vi "meTEC_Set_ID 50002_Live Set Voltage.vi"(6 "Instance (1)":u8=1, 8 "error in (no error)":errorcluster, 9 "TEC Configuration_IN":T1={"VISA resource name"="", "Device Address"=2}, 10 "Sequence No.":u16=5552, 11 "Live Set Voltage [V]":dbl) -> (0 "error out":errorcluster, 1 "TEC Configuration_OUT":T1={"VISA resource name"="", "Device Address"=2}, 3 "Serial Message_Read":string)   [LabVIEW 2023]
uses:
  TypeDefs/meTEC_Configuration.ctl
panel:
  # "--- Inputs ---"
  # "--- Outputs ---"
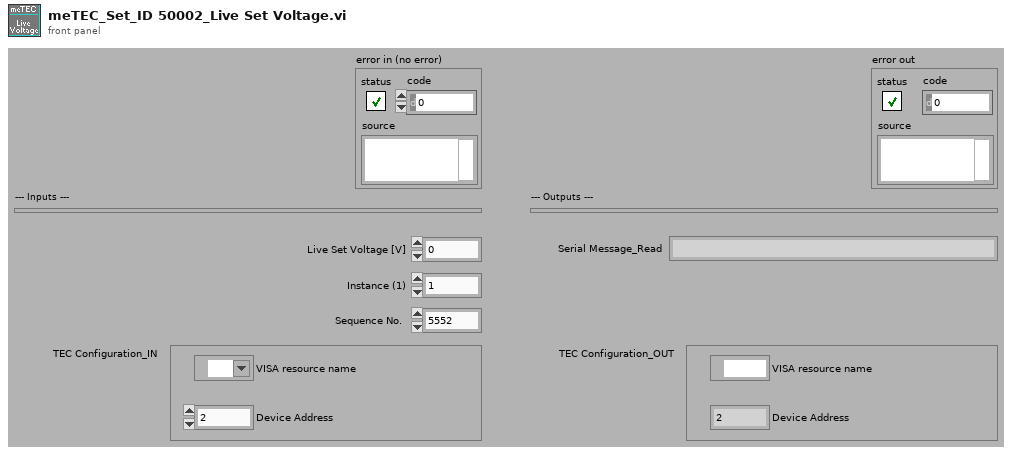
[diagram p1: front panel]
types:
  T1 = typedef "meTEC_Configuration.ctl" = cluster{"VISA resource name":refnum<visa-resource-name>, "Device Address":u16}
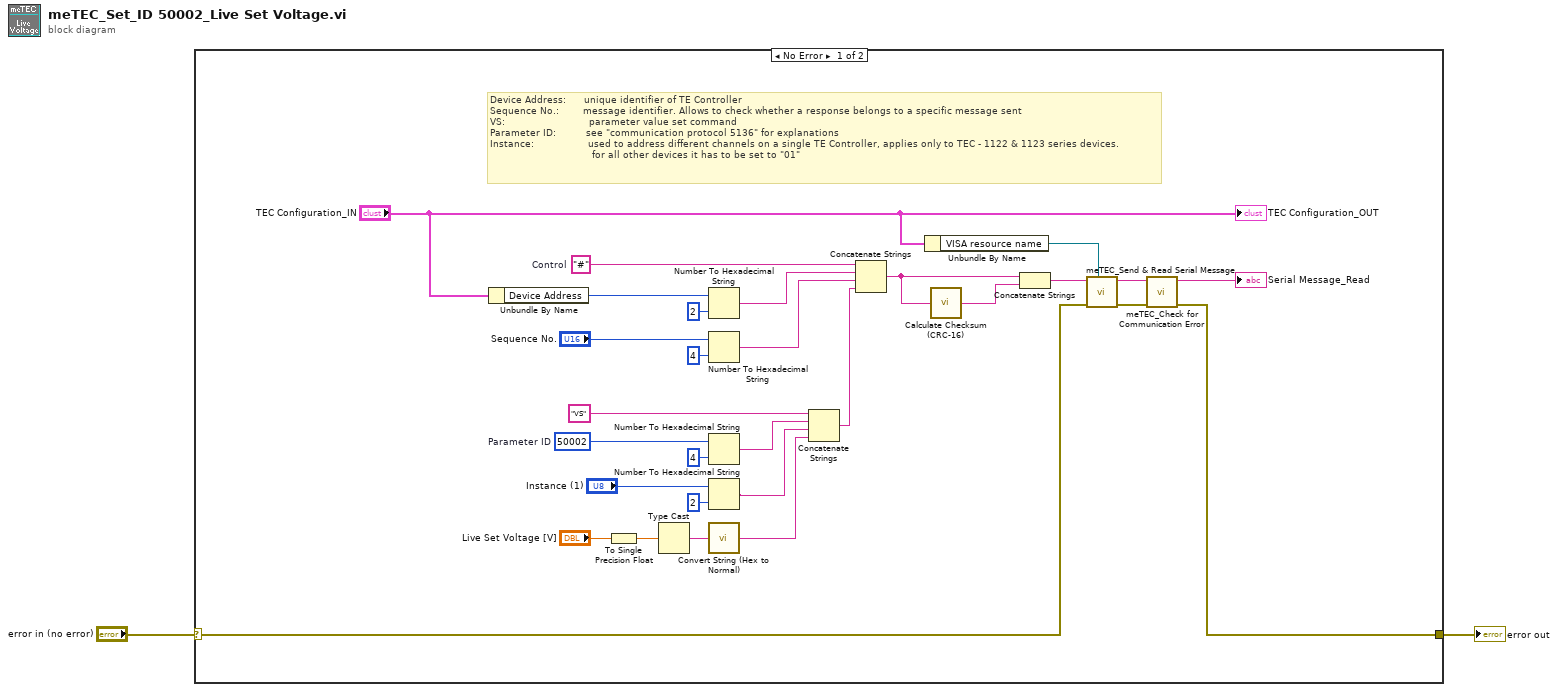
[diagram p0: block diagram]
diagram:
  n1 = case shown="No Error" "error in (no error)" {
    selector: "error in (no error)" -> [w15 w32]
    tunnel: [w5 w32] -> w2
    frame No Error {
      w23 = "#"  # Control
      w30 = 50002  # Parameter ID
      # "Device Address:      unique identifier of TE Controller\nSequence No.:        message identifier. Allows to check whether a response belongs to a specific message sent \nVS:                            parameter value set command\nParameter ID:          see \"communication protocol 5136\" for explanations\nInstance:                  used to address different channels on a single TE Controller, applies only to TEC - 1122 & 1123 series devices.\n                                  for all other devices it has to be set to \"01\""
      n2 = Unbundle By Name("TEC Configuration_IN") -> ("Device Address"=w10:u16)
      n3 = To Single Precision Float(number="Live Set Voltage [V]") -> (single precision float=w6:sgl)
      n4 = Type Cast(x=w6) -> (*(type *) &x=w26:string)  [unwired: 1 in]
      n5 = Number To Hexadecimal String(1:i16 2 ("width (-)"), 2:w10) -> (0:w18:string)
      n6 = Number To Hexadecimal String(1:i16 4 ("width (-)"), 2:"Sequence No.") -> (0:w22:string)
      n7 = Number To Hexadecimal String(1:i16 4 ("width (-)"), 2:w30) -> (0:w28:string)
      n8 = Number To Hexadecimal String(1:i16 2 ("width (-)"), 2:"Instance (1)") -> (0:w11:string)
      n9 = call "Convert String (Hex to Normal).vi"("Hex String"=w26) -> ("Normal String"=w27:string)  [unwired: 1 in]
      n10 = Concatenate Strings("VS", w28, w11, w27) -> (w17:string)
      n11 = Concatenate Strings(w23, w18, w22, w17) -> (w21:string)
      n12 = Unbundle By Name("TEC Configuration_IN") -> ("VISA resource name"=w13:refnum<visa-resource-name>)
      n13 = call "Calculate Checksum (CRC-16).vi"("Message"=w21) -> ("CRC [String]"=w20:string)  [unwired: 1 in]
      n14 = Concatenate Strings(w21, w20) -> (w16:string)
      n15 = call "meTEC_Send & Read Serial Message.vi"("VISA resource name"=w13, "error in (no error)"=w15, "Serial Message"=w16) -> ("error out"=w14:errorcluster, "Serial Message_Read"=w4:string)  [unwired: 7 in]
      n16 = call "meTEC_Check for Communication Error.vi"("error in (no error)"=w14, "Serial Message_IN"=w4) -> ("error out"=w5:errorcluster, "Serial Message_OUT"=→"Serial Message_Read":string)  [unwired: 8 in]
      "TEC Configuration_OUT" <- "TEC Configuration_IN"
    }
    frame Error {
    }
  }
  "error out" <- w2
